vi "Pre Launch Init.vi"(11 "Measure Object in":refnum<class "Measure Object.lvclass">) -> (0 "error out":errorcluster, 3 "Measure Object out":refnum<class "Measure Object.lvclass">)   [LabVIEW 2015, in "Measure Object.lvclass"]
doc: "(<B>Filename</B>: Actor Framework.lvlib:Actor.lvclass:Pre Launch Init.vi)\n\nDefines behavior that occurs after the Launch Nested Actor method is invoked but before the actor's Actor Core method begins running.\n\nBy default, this method does nothing. A descendant class may override it to define behavior."
uses:
  Measure Object.lvclass
  Measure Object.lvclass/Measure Object.ctl
  <vilib>/ActorFramework/Actor/Actor.lvclass
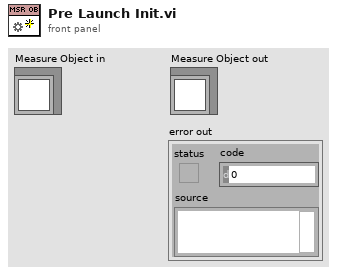
[diagram p1: front panel]
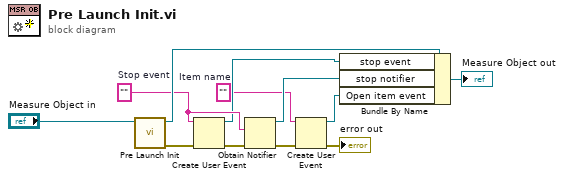
[diagram p0: block diagram]
diagram:
  w2 = ""  # Item name
  w10 = ""  # Stop event
  n1 = call-parent "Pre Launch Init.vi"("Actor in"="Measure Object in") -> ("error out"=w8:errorcluster, "Actor out"=w12:refnum<class "Measure Object.lvclass">)  [unwired: 9 in]
  n2 = Create User Event(user event datatype=w10, error in=w8) -> (user event=w6:refnum<user-event>, error out=w9:errorcluster)
  n3 = Obtain Notifier(notification data type=w10, error in (no error)=w9) -> (notifier out=w5:refnum<notifier>, error out=w4:errorcluster)  [unwired: 2 in, 1 out]
  n4 = Create User Event(user event datatype=w2, error in=w4) -> (user event=w1:refnum<user-event>, error out=→"error out":errorcluster)
  n5 = Bundle By Name(cluster=w12, "stop event"=w6, "stop notifier"=w5, "Open item event"=w1) -> (→"Measure Object out":refnum<class "Measure Object.lvclass">)
